vi "SERIAL_ProcessLoop.vi"() -> ()   [LabVIEW 2014, in "navX-MXP IMU.lvlib"]
uses:
  navX-MXP IMU.lvlib
  COMMON/TypeDefs/navX Device TypeDef.ctl
  COMMON/TypeDefs/Value TypeDefs/navX Interface Protocol.ctl
  <vilib>/Rock Robotics/WPI/SPI/WPI_SPIDevRef.ctl
  <vilib>/Rock Robotics/SystemInterfaces/Typedef/FPGA_TypedefDigitalModule.ctl
  <vilib>/Rock Robotics/SystemInterfaces/spilib/spi_bus.ctl
  <vilib>/Rock Robotics/WPI/I2C/WPI_I2CDevRef.ctl
  <vilib>/Rock Robotics/SystemInterfaces/i2clib/i2c_bus.ctl
  <vilib>/Rock Robotics/WPI/SerialPort/WPI_SerialPortRef.ctl
  COMMON/TypeDefs/Data TypeDefs/navX Board Information.ctl
  COMMON/TypeDefs/Value TypeDefs/navX NAVX_BOARD_CAPABILITY.ctl
  COMMON/TypeDefs/Value TypeDefs/navX NAVX_BOARD_YAW_AXIS.ctl
  COMMON/TypeDefs/Data TypeDefs/navX Status Data.ctl
  COMMON/TypeDefs/Value TypeDefs/navX NAVX_OP_STATUS.ctl
  COMMON/TypeDefs/Value TypeDefs/navX NAVX_CAL_STATUS.ctl
  COMMON/TypeDefs/Value TypeDefs/navX NAVX_SENSOR_STATUS.ctl
  COMMON/TypeDefs/Data TypeDefs/navX Offsets Data.ctl
  COMMON/TypeDefs/Value TypeDefs/navX Update Rate.ctl
  COMMON/TypeDefs/Value TypeDefs/navX Serial Mode.ctl
  <vilib>/Platform/TimedLoop/XDataNode/timing_clust.ctl
  <vilib>/Platform/TimedLoop/XDataNode/nitl_modes.ctl
  <vilib>/Platform/TimedLoop/XDataNode/wakeup.ctl
  COMMON/TypeDefs/Value TypeDefs/navX Device Registers.ctl
  <vilib>/Rock Robotics/SystemInterfaces/Utilities/FPGA_UtilitiesRead LocalTime.vi
  <vilib>/platform/TimedLoop/XDataNode/XDataNode.xnode
  <vilib>/Platform/TimedLoop/XDataNode/XDNodeRunTimeDep.lvlib
panel:
  in  "navX Device TypeDef":T1={"navX Interface Protocol"=enum."SPI", "navX Interface Protocol TypeDefs"={"SPIDevRef"={"DevStatus"={"status"=FALSE, "code"=0, "source"=""}, "Handle"=0, "Controller"=enum."Controller 1", "SPI Bus"=enum."SPI On-Board, CS0"}, "I2CDevRef"={"DevStatus"={"status"=FALSE, "code"=0, "source"=""}, "Controller"=enum."Controller 1", "Device Address"=0, "Handle"=0, "I2C Bus"=enum."Invalid"}, "SerialPortRef"={"DevStatus"={"status"=FALSE, "code"=0, "source"=""}, "Serial Port Name"=""}}, "navX System Information"={"Board Information"={"WhoAmI (50 | 0x32)"=0, "Board Revision"=0, "Firmware Major Version"=0, "Firmware Minor Version"=0, "NAVX_BOARD_CAPABILITY"={"OMNIMOUNT"=FALSE, "YAW_RESET"=FALSE, "VEL_AND_DISP"=FALSE}, "NAVX_BOARD_YAW_AXIS"={"BOARD_YAW_AXIS_UP"=FALSE, "BOARD_YAW_AXIS"=0}}, "Status"={"Update Rate Hz"=0, "Accelerometer Full-Scale Range"=0, "Gyro Full-Scale Range"=0, "NAVX_OP_STATUS"=0, "NAVX_CAL_STATUS"=0, "NAVX_SELFTEST_STATUS"=0, "NAVX_SENSOR_STATUS"={"MOVING"=FALSE, "YAW_STABLE"=FALSE, "MAG_DISTURBANCE"=FALSE, "ALTITUDE_VALID"=FALSE, "SEALEVEL_PRESS_SET"=FALSE, "FUSED_HEADING_VALID"=FALSE}}, "Offsets"={"Yaw"=0.0, "Quat W"=0.0, "Quat X"=0.0, "Quat Y"=0.0, "Quat Z"=0.0}, "LastSampleTimestamp"=0.0, "LastSampleValid"=FALSE}, "navX Common Information"={"Update Rate (4Hz-60Hz)"=50, "refnum name"="", "error"={"status"=FALSE, "code"=0, "source"=""}, "LastFPGATimestamp"=0.0, "Reboot Detected"=FALSE}, "Serial Protocol Extra"={"Loop VI Refnum"=refnum, "Nav6Mode (YPR)"=enum."Raw"}} {"navX Common Information"."Update Rate (4Hz-60Hz)" min=4 max=60 step=1; "navX System Information"."Status"."NAVX_OP_STATUS" items=["INITIALIZING", "SELFTEST_IN_PROGRESS", "ERROR", "IMU_AUTOCAL_IN_PROGRESS", "NORMAL"]; "navX System Information"."Status"."NAVX_CAL_STATUS" items=["IMU_CAL_STATE_MASK"=3, "IMU_CAL_INPROGRESS"=0, "IMU_CAL_ACCUMULATE"=1, "IMU_CAL_COMPLETE"=2, "MAG_CAL_COMPLETE"=4, "BARO_CAL_COMPLETE"=8]; "navX Interface Protocol TypeDefs"."I2CDevRef"."Device Address" format="%.0x"}
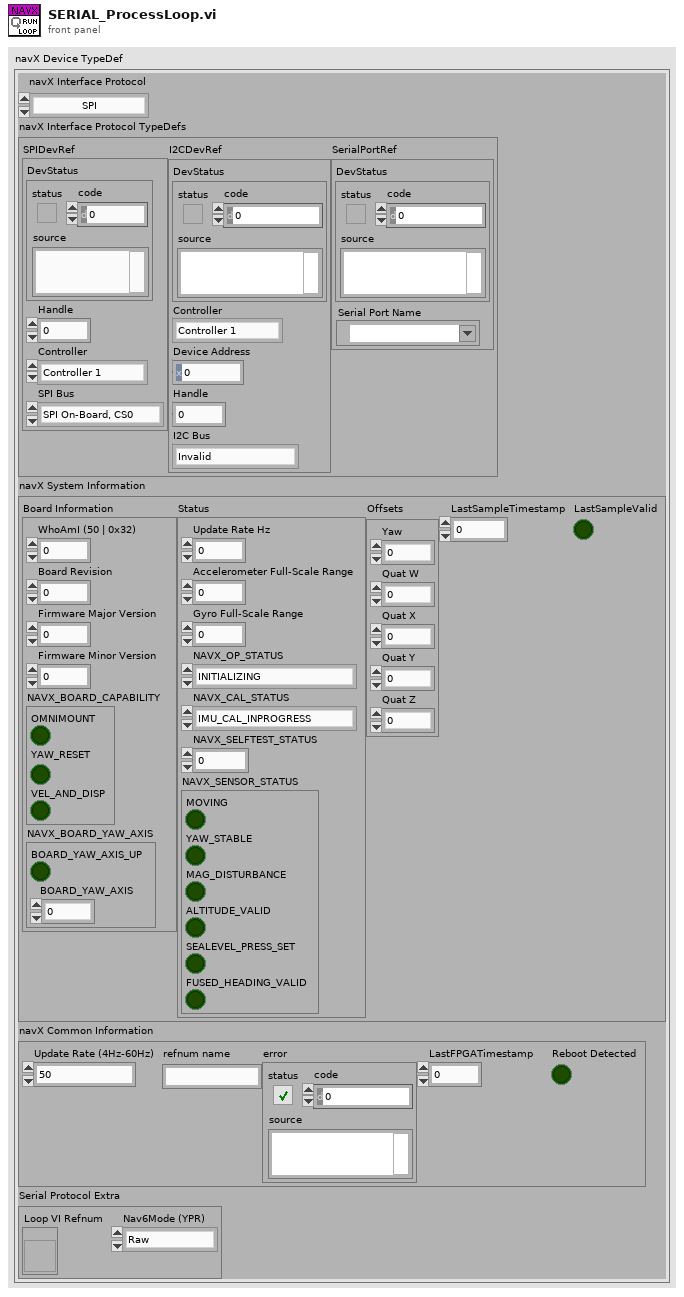
[diagram p1: front panel]
types:
  T1 = typedef "navX-MXP IMU.lvlib/navX Device TypeDef.ctl" = cluster{"navX Interface Protocol":T2, "navX Interface Protocol TypeDefs":cluster{"SPIDevRef":T3, "I2CDevRef":T6, "SerialPortRef":T8}, "navX System Information":cluster{"Board Information":T9, "Status":T12, "Offsets":T16, "LastSampleTimestamp":dbl, "LastSampleValid":bool}, "navX Common Information":cluster{"Update Rate (4Hz-60Hz)":T17, "refnum name":string, "error":errorcluster, "LastFPGATimestamp":dbl, "Reboot Detected":bool}, "Serial Protocol Extra":cluster{"Loop VI Refnum":refnum<vi>, "Nav6Mode (YPR)":T18}}
  T2 = typedef "navX-MXP IMU.lvlib/navX Interface Protocol.ctl" = enum16{"SPI", "I2C", "SERIAL"}
  T3 = typedef "WPI_SPIDevRef.ctl" = cluster{"DevStatus":errorcluster, "Handle":i32, "Controller":T4, "SPI Bus":T5}
  T4 = typedef "FPGA_TypedefDigitalModule.ctl" = enum16{"Controller 1"}
  T5 = typedef "spi_bus.ctl" = enum16{"SPI On-Board, CS0", "SPI On-Board, CS1", "SPI On-Board, CS2", "SPI On-Board, CS3", "SPI MXP", "Invalid"}
  T6 = typedef "WPI_I2CDevRef.ctl" = cluster{"DevStatus":errorcluster, "Controller":T4, "Device Address":u8, "Handle":i32, "I2C Bus":T7}
  T7 = typedef "i2c_bus.ctl" = enum16{"I2C On-Board", "I2C MXP", "Invalid"}
  T8 = typedef "WPI_SerialPortRef.ctl" = cluster{"DevStatus":errorcluster, "Serial Port Name":refnum<visa-resource-name>}
  T9 = typedef "navX-MXP IMU.lvlib/navX Board Information.ctl" = cluster{"WhoAmI (50 | 0x32)":u8, "Board Revision":u8, "Firmware Major Version":u8, "Firmware Minor Version":u8, "NAVX_BOARD_CAPABILITY":T10, "NAVX_BOARD_YAW_AXIS":T11}
  T10 = typedef "navX-MXP IMU.lvlib/navX NAVX_BOARD_CAPABILITY.ctl" = cluster{"OMNIMOUNT":bool, "YAW_RESET":bool, "VEL_AND_DISP":bool}
  T11 = typedef "navX-MXP IMU.lvlib/navX NAVX_BOARD_YAW_AXIS.ctl" = cluster{"BOARD_YAW_AXIS_UP":bool, "BOARD_YAW_AXIS":u8}
  T12 = typedef "navX-MXP IMU.lvlib/navX Status Data.ctl" = cluster{"Update Rate Hz":u8, "Accelerometer Full-Scale Range":u8, "Gyro Full-Scale Range":u16, "NAVX_OP_STATUS":T13, "NAVX_CAL_STATUS":T14, "NAVX_SELFTEST_STATUS":u8, "NAVX_SENSOR_STATUS":T15}
  T13 = typedef "navX-MXP IMU.lvlib/navX NAVX_OP_STATUS.ctl" = u8
  T14 = typedef "navX-MXP IMU.lvlib/navX NAVX_CAL_STATUS.ctl" = u8
  T15 = typedef "navX-MXP IMU.lvlib/navX NAVX_SENSOR_STATUS.ctl" = cluster{"MOVING":bool, "YAW_STABLE":bool, "MAG_DISTURBANCE":bool, "ALTITUDE_VALID":bool, "SEALEVEL_PRESS_SET":bool, "FUSED_HEADING_VALID":bool}
  T16 = typedef "navX-MXP IMU.lvlib/navX Offsets Data.ctl" = cluster{"Yaw":dbl, "Quat W":dbl, "Quat X":dbl, "Quat Y":dbl, "Quat Z":dbl}
  T17 = typedef "navX-MXP IMU.lvlib/navX Update Rate.ctl" = u8
  T18 = typedef "navX-MXP IMU.lvlib/navX Serial Mode.ctl" = enum16{"Raw", "Processed"}
  T19 = typedef "XDNodeRunTimeDep.lvlib/timing_clust.ctl" = cluster{"Expected End [f-1]":u64, "Actual End [f-1]":u64, "Finished Late? [f-1]":bool, "Expected End [i-1]":u64, "Actual End [i-1]":u64, "Finished Late? [i-1]":bool, "Expected Start [i]":u64, "Actual Start [i]":u64, "Expected Start [f]":u64, "Actual Start [f]":u64, "Source Name":string, "Structure Name":string, "Period":i64, "Deadline":i64, "Offset":i64, "Start":i64, "Priority":i32, "Timeout":i32, "Mode":T20, "Wakeup Reason":T21, "Error":errorcluster, "Source Type":string, "Secondary Source Type":string, "Global End Time":u64, "Global Start Time":u64, "Frame Duration":u64, "Iteration Duration":u64, "Assigned CPU":i32, "I/O Scan Engine Mode":u32}
  T20 = typedef "XDNodeRunTimeDep.lvlib/nitl_modes.ctl" = enum32{"No Change", "Process missed periods, maintain original phase", "Discard missed periods, maintain original phase", "Process missed periods, ignore original phase", "Discard missed periods, ignore original phase"}
  T21 = typedef "XDNodeRunTimeDep.lvlib/wakeup.ctl" = enum32{"Normal", "Aborted", "Asynchronous wakeup", "Timing source error", "Timed loop error", "Timeout"}
  T22 = typedef "navX-MXP IMU.lvlib/navX Device Registers.ctl" = u8
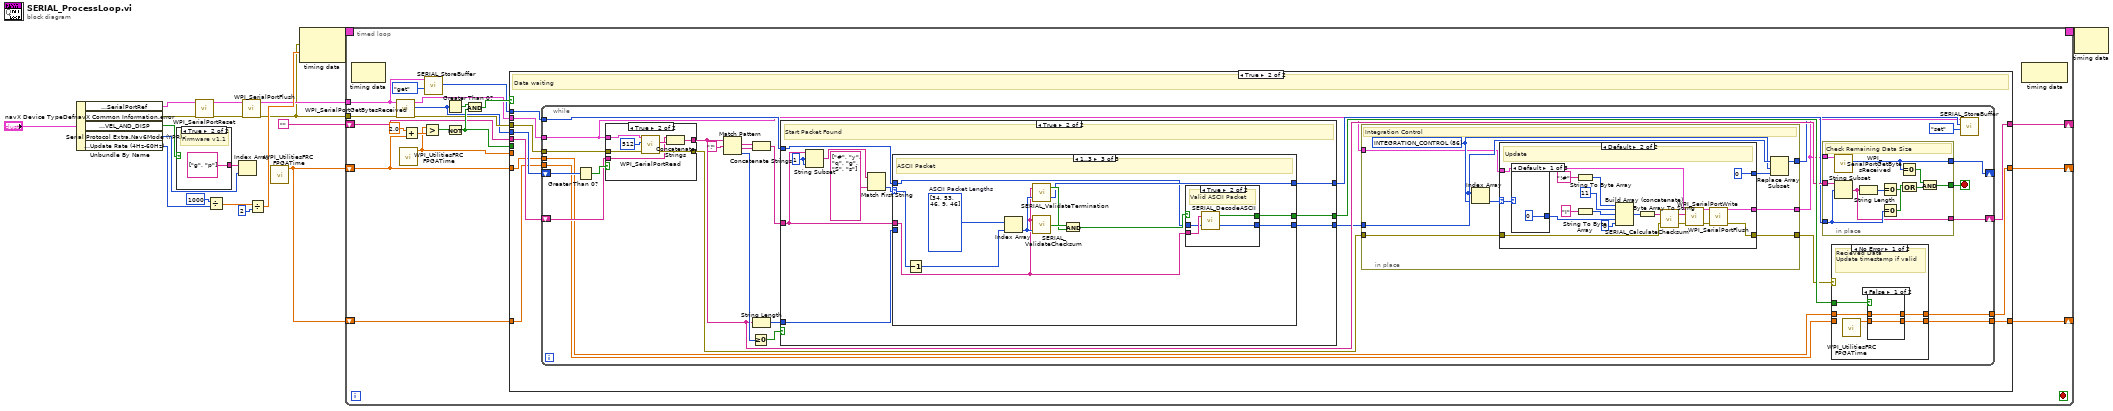
[diagram p0: block diagram]
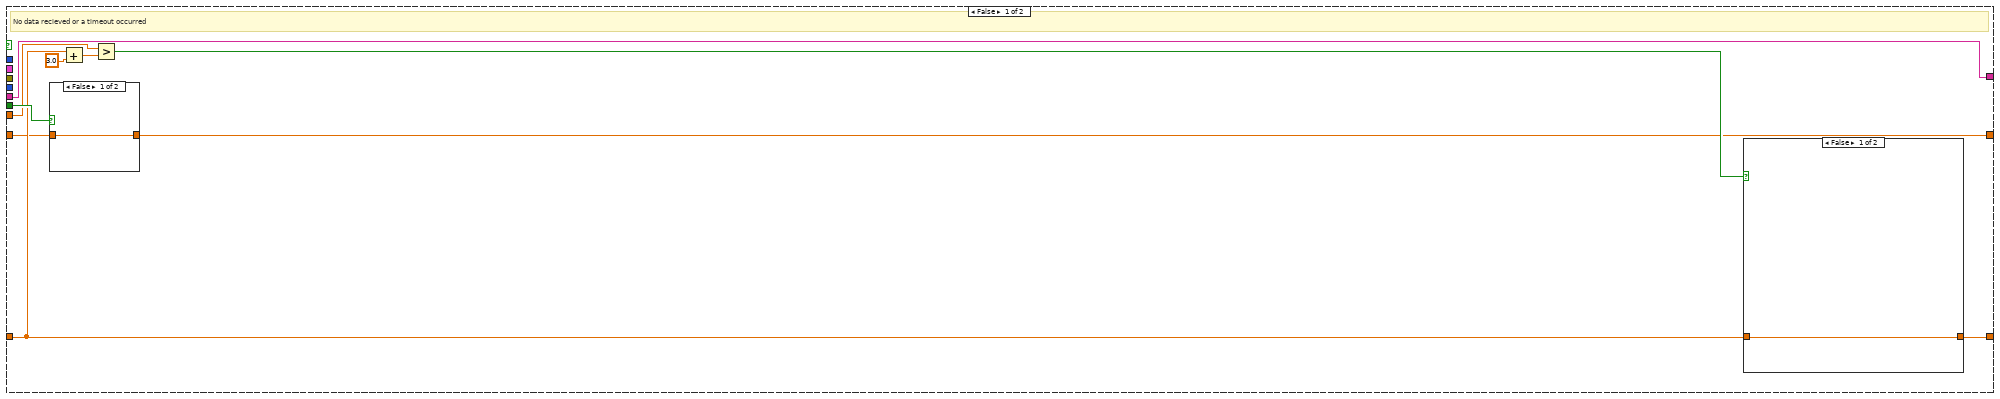
[diagram p2: hidden frame]
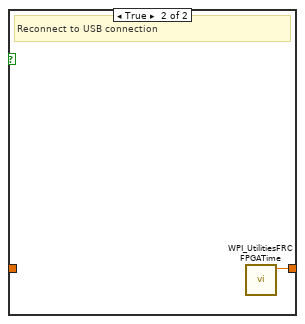
[diagram p3: hidden frame]
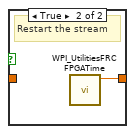
[diagram p4: hidden frame]
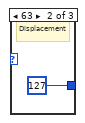
[diagram p6: hidden frame]
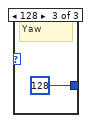
[diagram p7: hidden frame]
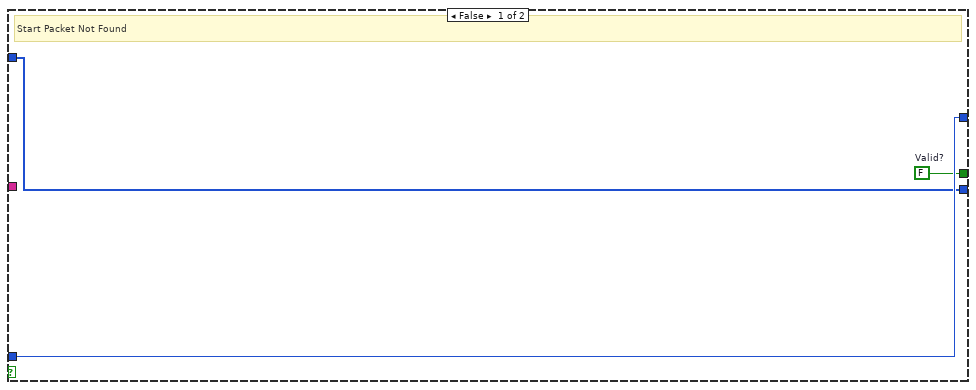
[diagram p8: hidden frame]
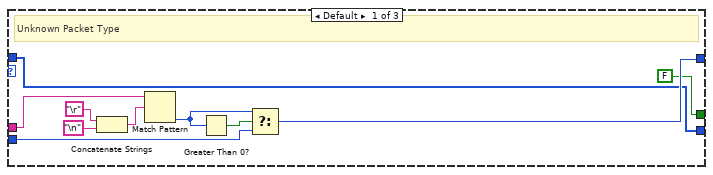
[diagram p9: hidden frame]
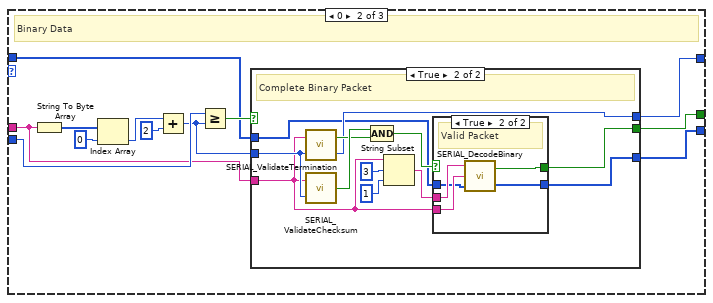
[diagram p10: hidden frame]
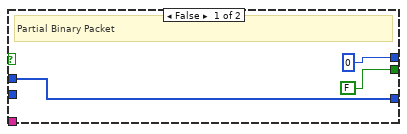
[diagram p11: hidden frame]
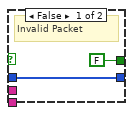
[diagram p12: hidden frame]
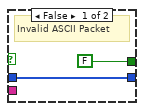
[diagram p13: hidden frame]
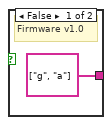
[diagram p17: hidden frame]
diagram:
  n1 = Unbundle By Name("navX Device TypeDef") -> ("navX Interface Protocol TypeDefs.SerialPortRef"=w17:T8, "navX Common Information.error"=w18:errorcluster, "navX System Information.Board Information.NAVX_BOARD_CAPABILITY.VEL_AND_DISP"=w9:bool, "Serial Protocol Extra.Nav6Mode (YPR)"=w8:T18, "navX Common Information.Update Rate (4Hz-60Hz)"=w7:T17)
  n2 = case shown="True" w9 {
    tunnel: [string[] ["g", "a"] string[] ["g", "p"]] -> w19
    frame False {
      # "Firmware v1.0"
    }
    frame True {
      # "Firmware v1.1"
    }
  }
  n3 = call <vilib>:"WPI_SerialPortReset.vi"("error in (no error)"=w18, "SerialPortRef"=w17) -> ("error out"=w16:errorcluster, "SerialPortRef"=w15:T8)  [unwired: 8 in]
  n4 = Divide(x=1000, y=w7) -> (x/y=w11:dbl)
  n5 = Index Array(array=w19, index=w8) -> ()  [unwired: 1 out]
  n6 = call <vilib>:"WPI_SerialPortFlush.vi"("error in (no error)"=w16, "SerialPortRef"=w15) -> ("error out"=w1:errorcluster, "SerialPortRef"=w2:T8)  [unwired: 8 in]
  n7 = Divide(x=w11, y=2) -> (x/y=w6:dbl)
  n8 = call <vilib>:"WPI_UtilitiesFRC FPGATime.vi"() -> ("FPGA Time"=w5:dbl)  [unwired: 10 in, 1 out]
  n9 = node-c288(w1, w6) -> (w14:T19)
  n10 = timed-loop {
    timing: w14 -> [_]
    timing-out: [_] -> w13
    shift-right: [w33] -> _
    shift-left: w5 -> [w31]
    shift-right: [w32] -> _
    shift-left: w5 -> [w35]
    shift-right: [w30] -> _
    shift-left: "" -> [w29]
    tunnel: w2 -> [w22]
    tunnel: w1 -> [w28]
    stop <- _ stop-if-true
    n11 = node-c288() -> ()  [unwired: 1 in, 1 out]
    n12 = call <vilib>:"WPI_SerialPortGetBytesReceived.vi"("error in (no error)"=w28, "SerialPortRef"=w22) -> ("error out"=w27:errorcluster, "Bytes at Port"=w26:u32, "SerialPortRef"=w25:T8)  [unwired: 7 in]
    n13 = call <vilib>:"WPI_UtilitiesFRC FPGATime.vi"() -> ("FPGA Time"=w34:dbl)  [unwired: 10 in, 1 out]
    n14 = Add(x=2.0, y=w31) -> (x+y=w40:dbl)
    n15 = Greater?(x=w34, y=w40) -> (0:w39:bool)
    n16 = call "SERIAL_StoreBuffer.vi"("Access Type"=enum16{"set", "get", "delete"}."get", "SerialPortRef"=w22) -> ("navX Data"=w24:u8[])  [unwired: 7 in, 2 out]
    n17 = Greater Than 0?(x=w26) -> (x > 0?=w38:bool)
    n18 = Not(x=w39) -> (.not. x?=w36:bool)
    n19 = Compound Arithmetic op=AND(w38, w36) -> (w37:bool)
    n20 = case shown="True" w37 {
      tunnel: w36 -> [w51 _]
      tunnel: w35 -> [w44 w58]
      tunnel: w34 -> [w48 _]
      tunnel: [w46 w60] -> w33
      tunnel: [w45 w57] -> w32
      tunnel: w31 -> [w43 w59]
      tunnel: [w42 w65] -> w30
      tunnel: w29 -> [w42 w64]
      tunnel: w27 -> [_ w63]
      tunnel: w26 -> [_ w62]
      tunnel: w25 -> [_ w61]
      tunnel: w24 -> [_ w56]
      frame False {
        # "No data recieved or a timeout occurred"
        n21 = case shown="False" w51 {
          tunnel: [w54 w55] -> w46
          tunnel: w43 -> [w54 _]
          frame False {
          }
          frame True {
            # "Restart the stream"
            n22 = call <vilib>:"WPI_UtilitiesFRC FPGATime.vi"() -> ("FPGA Time"=w55:dbl)  [unwired: 10 in, 1 out]
          }
        }
        n23 = Add(x=w44, y=3.0) -> (x+y=w49:dbl)
        n24 = Greater?(x=w48, y=w49) -> (0:w47:bool)
        n25 = case shown="False" w47 {
          tunnel: [w52 w53] -> w45
          tunnel: w44 -> [w52 _]
          frame False {
          }
          frame True {
            # "Reconnect to USB connection"
            n26 = call <vilib>:"WPI_UtilitiesFRC FPGATime.vi"() -> ("FPGA Time"=w53:dbl)  [unwired: 10 in, 1 out]
          }
        }
      }
      frame True {
        # "Data waiting"
        n27 = while {
          shift-right: [w75] -> w65
          shift-left: w64 -> [w91]
          tunnel: w63 -> [w92]
          tunnel: w61 -> [w69]
          tunnel: [w89] -> w60
          tunnel: w59 -> [w88]
          tunnel: w58 -> [w87]
          tunnel: [w86] -> w57
          shift-right: [w78] -> _
          shift-left: w62 -> [w94]
          tunnel: w56 -> [w73]
          stop <- w74 stop-if-true
          n28 = Greater Than 0?(x=w94) -> (x > 0?=w93:bool)
          n29 = case shown="True" w93 {
            tunnel: w69 -> [_ w233]
            tunnel: w92 -> [w226 w232]
            tunnel: [w226 w231] -> w68
            tunnel: w91 -> [w225 w228]
            tunnel: [w225 w227] -> w77
            frame False {
            }
            frame True {
              n30 = call <vilib>:"WPI_SerialPortRead.vi"("error in (no error)"=w232, "Num Bytes to Read"=u32 512, "SerialPortRef"=w233) -> ("error out"=w231:errorcluster, "Buffer"=w229:string)  [unwired: 6 in, 1 out]
              n31 = Concatenate Strings(w228, w229) -> (w227:string)
            }
          }
          n32 = Match Pattern(string=w77, regular expression="!") -> (match substring=w80:string, after substring=w82:string, offset past match=w90:i32)  [unwired: 1 in, 1 out]
          n33 = Greater Or Equal To 0?(x=w90) -> (x >= 0?=w85:bool)
          n34 = Concatenate Strings(w80, w82) -> (w79:string)
          n35 = String Length(string=w77) -> (length=w84:i32)
          n36 = case shown="True" w85 {
            tunnel: w84 -> [w142 w150]
            tunnel: [w142 w149] -> w76
            tunnel: [w141 w148] -> w83
            tunnel: w79 -> [_ w145]
            tunnel: [w140 w147] -> w71
            tunnel: w73 -> [w140 w143]
            frame False {
              w141 = FALSE  # Valid?
              # "Start Packet Not Found"
            }
            frame True {
              w146 = 1 ("offset (0)")
              # "Start Packet Found"
              n37 = String Subset(string=w145, offset (0)=w146, length (rest)=w146) -> (substring=w144:string)
              n38 = Match First String(2:string[] ["#", "y", "q", "g", "S", "s"], 3:w144) -> (0:w151:i32)  [unwired: 1 out]
              n39 = case shown="1..3" w151 {
                selector: w151 -> [_ _ w207]
                tunnel: w145 -> [w156 w167 w200]
                tunnel: w150 -> [w157 w171 _]
                tunnel: [w155 w168 w198] -> w149
                tunnel: [FALSE ("Valid?") w169 w201] -> w148
                tunnel: [w153 w164 w199] -> w147
                tunnel: w143 -> [w153 w163 w197]
                frame Default {
                  # "Unknown Packet Type"
                  n40 = Concatenate Strings("\r", "\n") -> (w160:string)
                  n41 = Match Pattern(string=w156, regular expression=w160) -> (offset past match=w158:i32)  [unwired: 1 in, 3 out]
                  n42 = Greater Than 0?(x=w158) -> (x > 0?=w159:bool)
                  n43 = Select(t=w158, s=w159, f=w157) -> (s? t:f=w155:i32)
                }
                frame 0 {
                  # "Binary Data"
                  n44 = String To Byte Array(string=w167) -> (unsigned byte array=w174:u8[])
                  n45 = Index Array(array=w174, index=0) -> (element=w173:u8)
                  n46 = Add(x=w173, y=u8 2) -> (x+y=w166:u8)
                  n47 = Greater Or Equal?(x=w171, y=w166) -> (x >= y?=w170:bool)
                  n48 = case shown="True" w170 {
                    tunnel: [FALSE w180] -> w169
                    tunnel: [0 w182] -> w168
                    tunnel: w167 -> [_ w181]
                    tunnel: w166 -> [_ w185]
                    tunnel: [w175 w179] -> w164
                    tunnel: w163 -> [w175 w178]
                    frame False {
                      # "Partial Binary Packet"
                    }
                    frame True {
                      # "Complete Binary Packet"
                      n49 = call "SERIAL_ValidateTermination.vi"("Expected Packet Length"=w185, "Content"=w181) -> ("Termination Offset"=w182:i32, "Valid?"=w184:bool)
                      n50 = call "SERIAL_ValidateChecksum.vi"("Expected Packet Length"=w185, "Content"=w181) -> ("Valid?"=w186:bool)
                      n51 = Compound Arithmetic op=AND(w186, w184) -> (w183:bool)
                      n52 = String Subset(string=w181, offset (0)=3, length (rest)=1 ("length (rest)")) -> (substring=w187:string)
                      n53 = case shown="True" w183 {
                        tunnel: w187 -> [_ w196]
                        tunnel: w181 -> [_ w195]
                        tunnel: [FALSE ("Valid?") w194] -> w180
                        tunnel: [w190 w193] -> w179
                        tunnel: w178 -> [w190 w192]
                        frame False {
                          # "Invalid Packet"
                        }
                        frame True {
                          # "Valid Packet"
                          n54 = call "SERIAL_DecodeBinary.vi"("navX Data"=w192, "Buffer"=w195, "Update Type"=w196) -> ("navX Data"=w193:u8[], "Valid?"=w194:bool)
                        }
                      }
                    }
                  }
                }
                frame 1..3 {
                  w208 = i32[] [34, 53, 46, 9, 46]  # ASCII Packet Lengths
                  # "ASCII Packet"
                  n55 = Decrement(x=w207) -> (x-1=w206:i32)
                  n56 = Index Array(array=w208, index=w206) -> (element=w205:i32)
                  n57 = call "SERIAL_ValidateTermination.vi"("Expected Packet Length"=w205, "Content"=w200) -> ("Termination Offset"=w198:i32, "Valid?"=w203:bool)
                  n58 = call "SERIAL_ValidateChecksum.vi"("Expected Packet Length"=w205, "Content"=w200) -> ("Valid?"=w204:bool)
                  n59 = Compound Arithmetic op=AND(w204, w203) -> (w202:bool)
                  n60 = case shown="True" w202 {
                    tunnel: [FALSE w214] -> w201
                    tunnel: w200 -> [_ w212]
                    tunnel: [w209 w213] -> w199
                    tunnel: w197 -> [w209 w211]
                    frame False {
                      # "Invalid ASCII Packet"
                    }
                    frame True {
                      # "Valid ASCII Packet"
                      n61 = call "SERIAL_DecodeASCII.vi"("navX Data"=w211, "Buffer"=w212) -> ("navX Data"=w213:u8[], "Valid?"=w214:bool)
                    }
                  }
                }
              }
            }
          }
          n62 = in-place {
            in-place-border: w71 -> [w102]
            in-place-border: [w99] -> w70
            in-place-border: [w98] -> w66
            in-place-border: w69 -> [w97]
            in-place-border: w68 -> [w96]
            in-place-border: [w95] -> w67
            w101 = T22 86 items=["WHOAMI"=0, "HW_REV"=1, "FW_VER_MAJOR"=2, "FW_VER_MINOR"=3, "UPDATE_RATE_HZ"=4, "ACCEL_FSR_G"=5, "GYRO_FSR_DPS"=6, "OP_STATUS"=8, "CAL_STATUS"=9, "SELFTEST_STATUS"=10, "CAPABILITY_FLAGS_L"=11, "CAPABILITY_FLAGS_H"=12, "SENSOR_STATUS"=16, "TIMESTAMP"=18, "YAW"=22, "PITCH"=24, "ROLL"=26, "HEADING"=28, "FUSED_HEADING"=30, "ALTITUDE_I"=32, "ALTITUDE_D"=34, "LINERA_ACC_X"=36, "LINERA_ACC_Y"=38, "LINERA_ACC_Z"=40, "QUAT_W"=42, "QUAT_X"=44, "QUAT_Y"=46, "QUAT_Z"=48, "MPU_TEMP_C"=50, "GYRO_X"=52, "GYRO_Y"=54, "GYRO_Z"=56, "ACC_X"=58, "ACC_Y"=60, "ACC_Z"=62, "MAG_X"=64, "MAG_Y"=66, "MAG_Z"=68, "PRESSURE_I"=70, "PRESSURE_D"=72, "PRESSURE_TEMP"=74, "YAW_OFFSET"=76, "QUAT_OFFSET_W"=78, "QUAT_OFFSET_X"=80, "QUAT_OFFSET_Y"=82, "QUAT_OFFSET_Z"=84, "INTEGRATION_CONTROL"=86, "VELOCITY_X"=88, "VELOCITY_Y"=92, "VELOCITY_Z"=96, "DISPLACMENT_X"=100, "DISPLACMENT_Y"=104, "DISPLACEMENT_Z"=108] ("Device Register")
            # "Integration Control"
            n63 = Index Array(array=w102, index=w101) -> (element=w103:u8)
            n64 = case shown="Default" w103 {
              selector: w103 -> [w106 w124]
              tunnel: [w106 0] -> w100
              tunnel: [w105 w110] -> w98
              tunnel: [w104 w109] -> w95
              tunnel: w97 -> [w105 w108]
              tunnel: w96 -> [w104 w107]
              frame 0 {
              }
              frame Default {
                # "Update"
                n65 = case shown="Default" w124 {
                  tunnel: [0 127 128] -> w117
                  frame Default {
                  }
                  frame 63 {
                    # "Displacement"
                  }
                  frame 128 {
                    # "Yaw"
                  }
                }
                n66 = String To Byte Array(string="!#") -> (unsigned byte array=w121:u8[])
                n67 = String To Byte Array(string="I" ("format string")) -> (unsigned byte array=w119:u8[])
                n68 = Build Array (concatenate)(w121, 11, w119, w117, 0) -> (w116:i32[])
                n69 = Byte Array To String(unsigned byte array=w116) -> (string=w115:string)
                n70 = call "SERIAL_CalculateChecksum.vi"("error in"=w107, "Content"=w115) -> ("error out"=w111:errorcluster, "Teminated Content"=w112:string)
                n71 = call <vilib>:"WPI_SerialPortWrite.vi"("error in (no error)"=w111, "Buffer"=w112, "SerialPortRef"=w108) -> ("error out"=w114:errorcluster, "SerialPortRef"=w113:T8)  [unwired: 6 in, 1 out]
                n72 = call <vilib>:"WPI_SerialPortFlush.vi"("error in (no error)"=w114, "SerialPortRef"=w113) -> ("error out"=w109:errorcluster, "SerialPortRef"=w110:T8)  [unwired: 8 in]
              }
            }
            n73 = Replace Array Subset(array=w102, new element=w100, index=w101) -> (w99:u8[])
          }
          n74 = in-place {
            in-place-border: w66 -> [w139]
            in-place-border: [w138] -> w78
            in-place-border: w77 -> [w137]
            in-place-border: w76 -> [w136]
            in-place-border: [w135] -> w75
            in-place-border: [w129] -> w74
            # "Check Remaining Data Size"
            n75 = call <vilib>:"WPI_SerialPortGetBytesReceived.vi"("SerialPortRef"=w139) -> ("Bytes at Port"=w138:u32)  [unwired: 8 in, 2 out]
            n76 = String Subset(string=w137, offset (0)=w136) -> (substring=w135:string)  [unwired: 1 in]
            n77 = String Length(string=w135) -> (length=w134:i32)
            n78 = Equal To 0?(x=w134) -> (x = 0?=w132:bool)
            n79 = Equal To 0?(x=w136) -> (x = 0?=w133:bool)
            n80 = Equal To 0?(x=w138) -> (x = 0?=w131:bool)
            n81 = Compound Arithmetic op=OR(w133, w132) -> (w130:bool)
            n82 = Compound Arithmetic op=AND(w131, w130) -> (w129:bool)
          }
          n83 = case shown="No Error" w67 {
            tunnel: [w219 w224] -> w89
            tunnel: w88 -> [w218 w224]
            tunnel: w87 -> [_ w223]
            tunnel: [w217 w223] -> w86
            tunnel: w83 -> [w215 _]
            frame No Error {
              # "Recieved Data\nUpdate timestamp if valid"
              n84 = call <vilib>:"WPI_UtilitiesFRC FPGATime.vi"() -> ("FPGA Time"=w216:dbl)  [unwired: 10 in, 1 out]
              n85 = case shown="False" w215 {
                tunnel: [w221 w222] -> w219
                tunnel: w218 -> [w221 _]
                tunnel: [w220 w222] -> w217
                tunnel: w216 -> [w220 w222]
                frame False {
                }
                frame True {
                }
              }
            }
            frame Error {
            }
          }
          n86 = call "SERIAL_StoreBuffer.vi"("Access Type"=enum16{"set", "get", "delete"}."set", "navX Data"=w70, "SerialPortRef"=w66) -> ()  [unwired: 6 in, 3 out]
        }
      }
    }
    n87 = node-c288() -> ()  [unwired: 1 in, 1 out]
  }
  n88 = node-c288(w13) -> ()  [unwired: 1 out]
